vi "GetParentInterfaces.vi"(0 "ClassReader in":refnum<class "ClassReader.lvclass">, 5 "error in (no error)":errorcluster) -> (14 "ClassReader out":refnum<class "ClassReader.lvclass">, 15 "ParentInterfaces":path[](array[path]), 19 "error out":errorcluster)   [LabVIEW 2020, in "ClassReader.lvclass"]
uses:
  <resource>/Framework/Providers/Open_GDS/ClassProviders/Provider_BaseClassInterface/ClassReader_class/ClassReader.lvclass
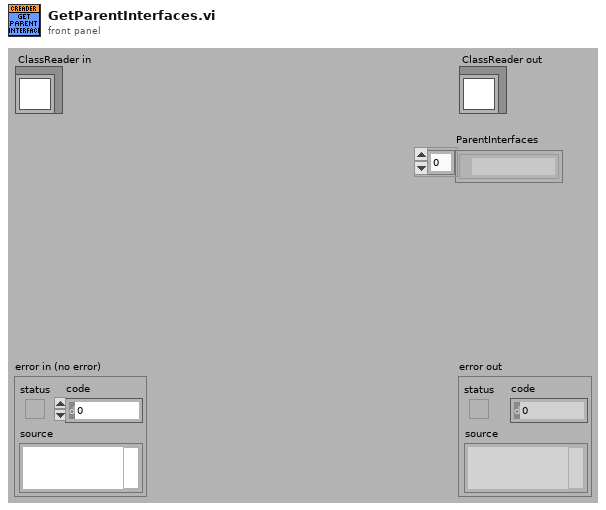
[diagram p1: front panel]
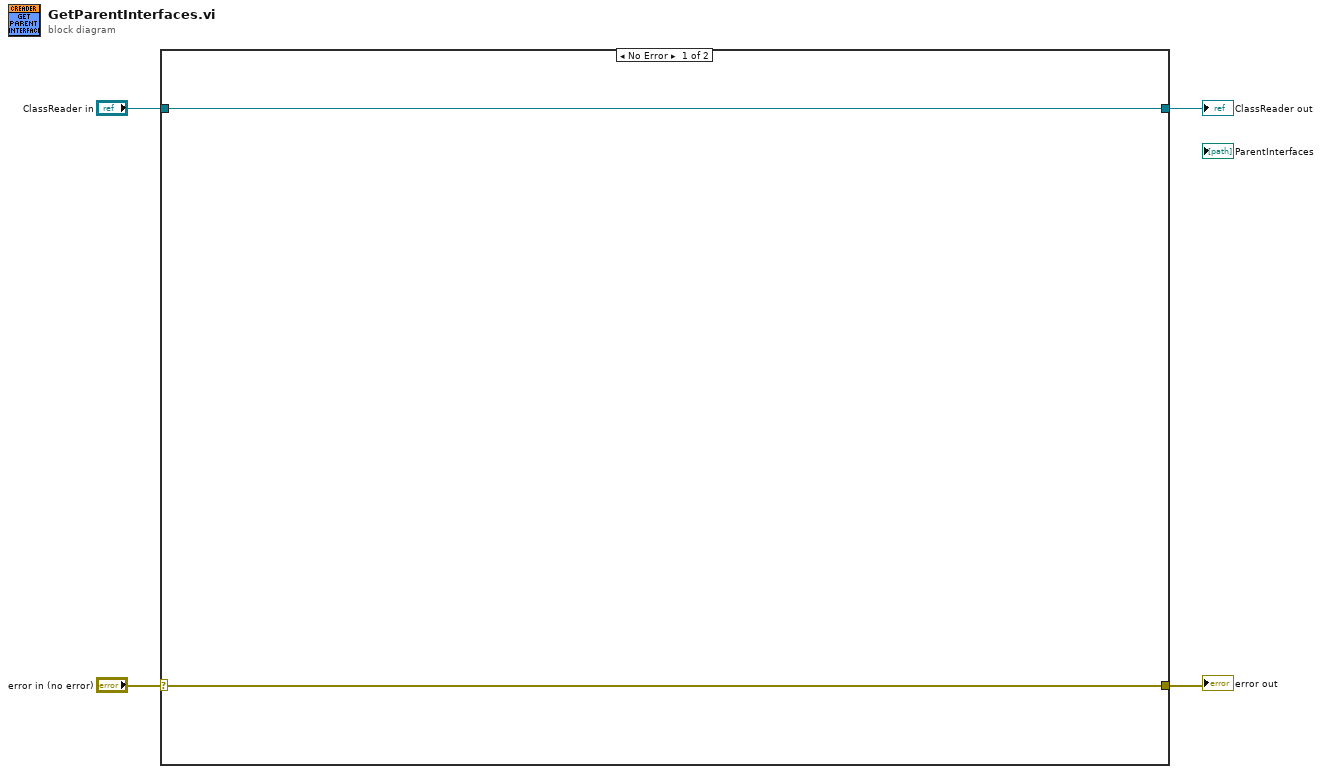
[diagram p0: block diagram]
diagram:
  n1 = case shown="No Error" "error in (no error)" {
    selector: "error in (no error)" -> [w5 w8]
    tunnel: [w5 w8] -> w3
    tunnel: [w6 w7] -> w1
    tunnel: "ClassReader in" -> [w6 w7]
    frame No Error {
    }
    frame Error {
    }
  }
  "error out" <- w3
  "ClassReader out" <- w1
